vi "设置电能表.vi"(3 "电能表参数":T1={"有功常数"=200, "无功常数"=3600000, "校验圈数"=5, "校验类型"=0, "S值计算次数"=5, "S值计算方法"=0}, 6 "脉冲输入口":u8, 7 "串口号":refnum<visa-resource-name>) -> (1 "应答":string)   [LabVIEW 2014]
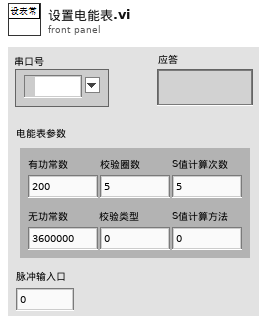
[diagram p1: front panel]
types:
  T1 = cluster{"有功常数":i32, "无功常数":i32, "校验圈数":i32, "校验类型":i32, "S值计算次数":i32, "S值计算方法":i32}
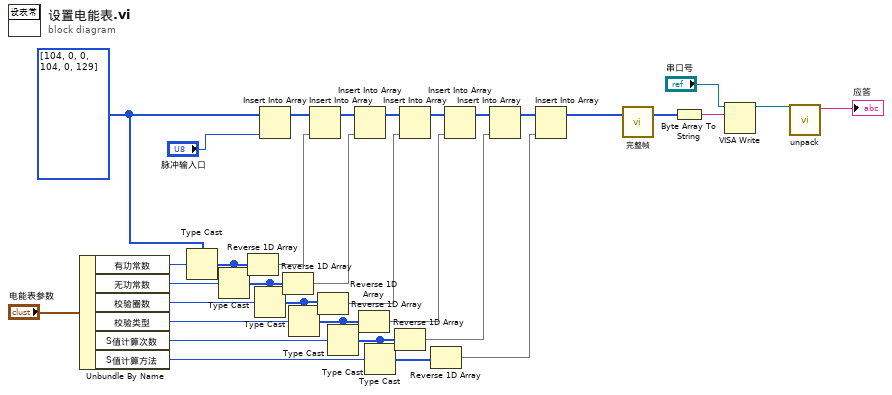
[diagram p0: block diagram]
diagram:
  w25 = u8[] [104, 0, 0, 104, 0, 129]
  n1 = Unbundle By Name("电能表参数") -> ("有功常数"=w30:i32, "无功常数"=w29:i32, "校验圈数"=w28:i32, "校验类型"=w24:i32, "S值计算次数"=w27:i32, "S值计算方法"=w26:i32)
  n2 = Type Cast(type=w25, x=w30) -> (*(type *) &x=w22:u8[])
  n3 = Type Cast(type=w22, x=w29) -> (*(type *) &x=w21:u8[])
  n4 = Reverse 1D Array(array=w22) -> (reversed array=w17:u8[])
  n5 = Type Cast(type=w21, x=w28) -> (*(type *) &x=w20:u8[])
  n6 = Insert Into Array(array=w25, new element="脉冲输入口") -> (w33:u8[])  [unwired: 1 in]
  n7 = Reverse 1D Array(array=w21) -> (reversed array=w16:u8[])
  n8 = Type Cast(type=w20, x=w24) -> (*(type *) &x=w19:u8[])
  n9 = Insert Into Array(array=w33, new element=w17) -> (w15:u8[])  [unwired: 1 in]
  n10 = Reverse 1D Array(array=w20) -> (reversed array=w10:u8[])
  n11 = Type Cast(type=w19, x=w27) -> (*(type *) &x=w18:u8[])
  n12 = Insert Into Array(array=w15, new element=w16) -> (w14:u8[])  [unwired: 1 in]
  n13 = Reverse 1D Array(array=w19) -> (reversed array=w9:u8[])
  n14 = Type Cast(type=w18, x=w26) -> (*(type *) &x=w23:u8[])
  n15 = Reverse 1D Array(array=w18) -> (reversed array=w8:u8[])
  n16 = Insert Into Array(array=w14, new element=w10) -> (w13:u8[])  [unwired: 1 in]
  n17 = Reverse 1D Array(array=w23) -> (reversed array=w7:u8[])
  n18 = Insert Into Array(array=w13, new element=w9) -> (w12:u8[])  [unwired: 1 in]
  n19 = Insert Into Array(array=w12, new element=w8) -> (w11:u8[])  [unwired: 1 in]
  n20 = Insert Into Array(array=w11, new element=w7) -> (w6:u8[])  [unwired: 1 in]
  n21 = call "完整帧.vi"("不完整帧"=w6) -> ("完整帧"=w1:u8[])  [unwired: 2 in]
  n22 = Byte Array To String(unsigned byte array=w1) -> (string=w2:string)
  n23 = VISA Write(VISA resource name="串口号", write buffer=w2) -> (VISA resource name out=w4:refnum<visa-resource-name>)  [unwired: 1 in, 2 out]
  n24 = call "unpack.vi"("串口号输入"=w4) -> ("应答"=→"应答":string)  [unwired: 5 in, 1 out]
